vi "STM32.DAC.vi"(6 "FileName":string, 7 "CMD":enum16{"Sine", "File", "Close Output"}(ring), 8 "Error In":errorcluster, 9 "AMP":u8, 10 "FREQ":u16, 11 "VISA_USB":refnum<visa-resource-name>) -> (0 "Error Out":errorcluster, 1 "Points":i32, 2 "命令数":u32, 3 "CMD List":string[](array[string]))   [LabVIEW 2012, in "Lib_UEL.ATE.lvlib" / "STM32-CoreBD.lvlib"]
uses:
  STM32-CoreBD.lvlib
  <vilib>/regexp/Match Regular Expression.xnode
panel:
  # "Version History\nV01,2014-4-30, 初始版本."
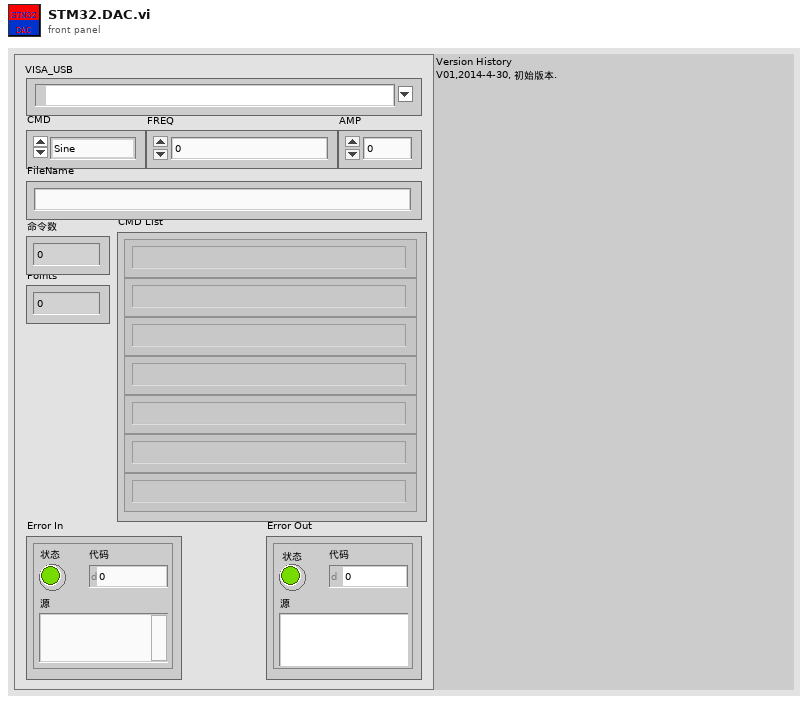
[diagram p1: front panel]
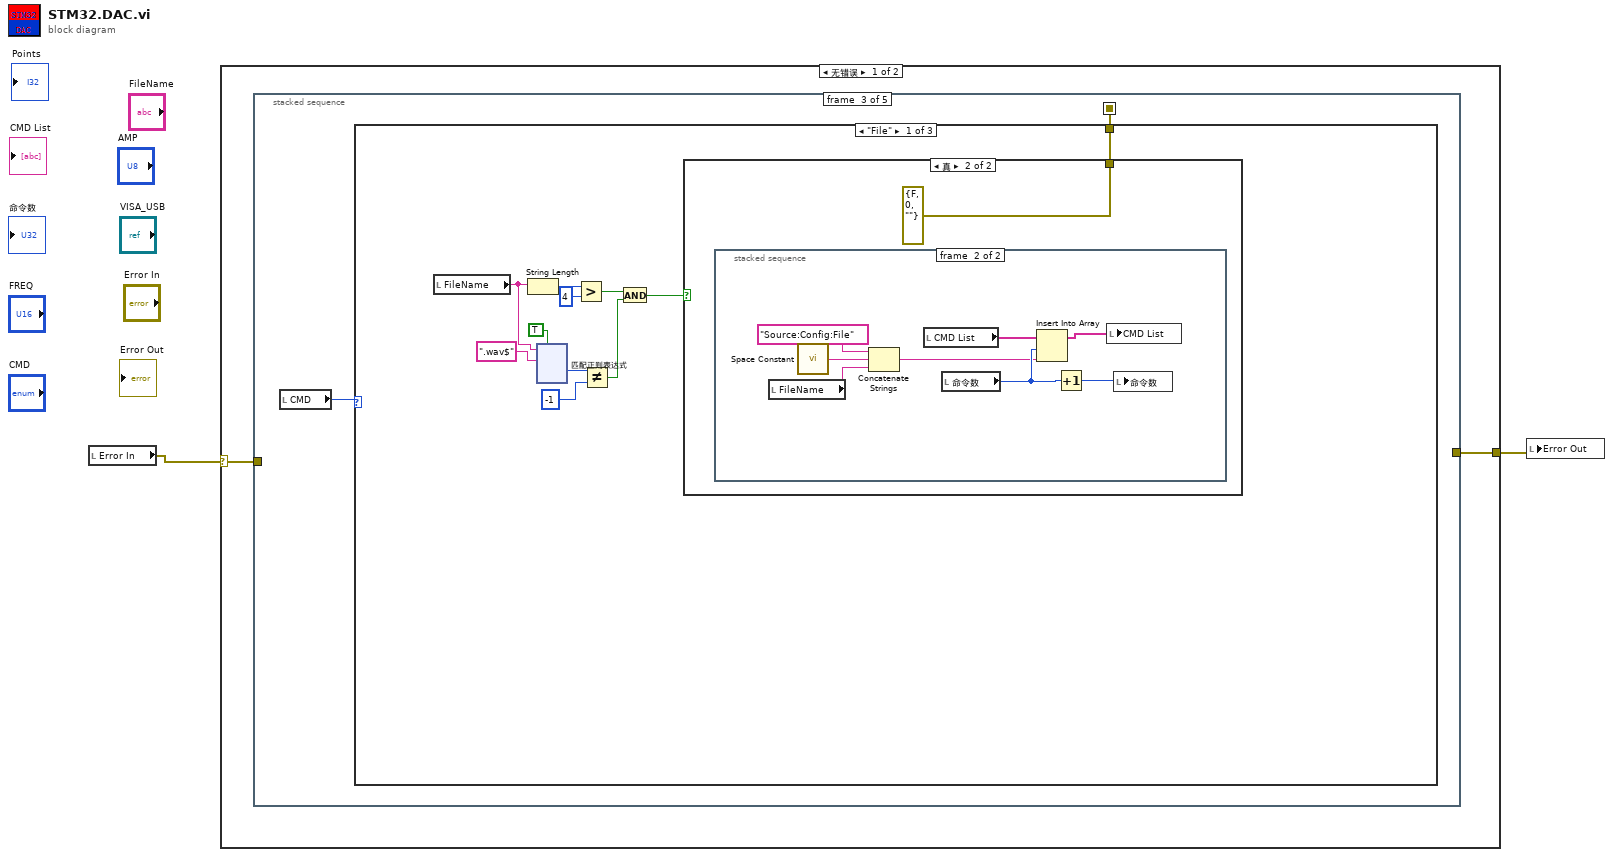
[diagram p0: block diagram]
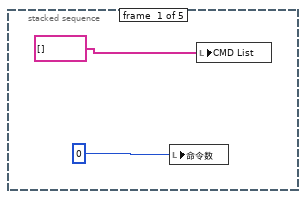
[diagram p2: hidden frame]
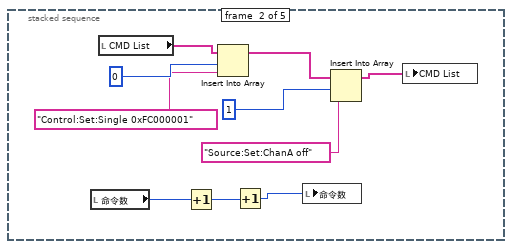
[diagram p3: hidden frame]
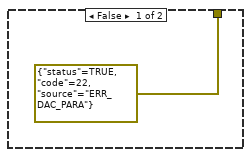
[diagram p4: hidden frame]
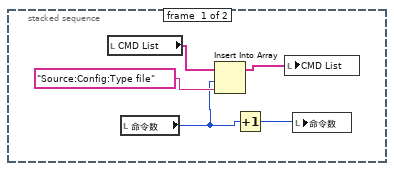
[diagram p5: hidden frame]
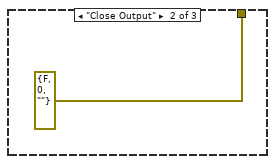
[diagram p6: hidden frame]
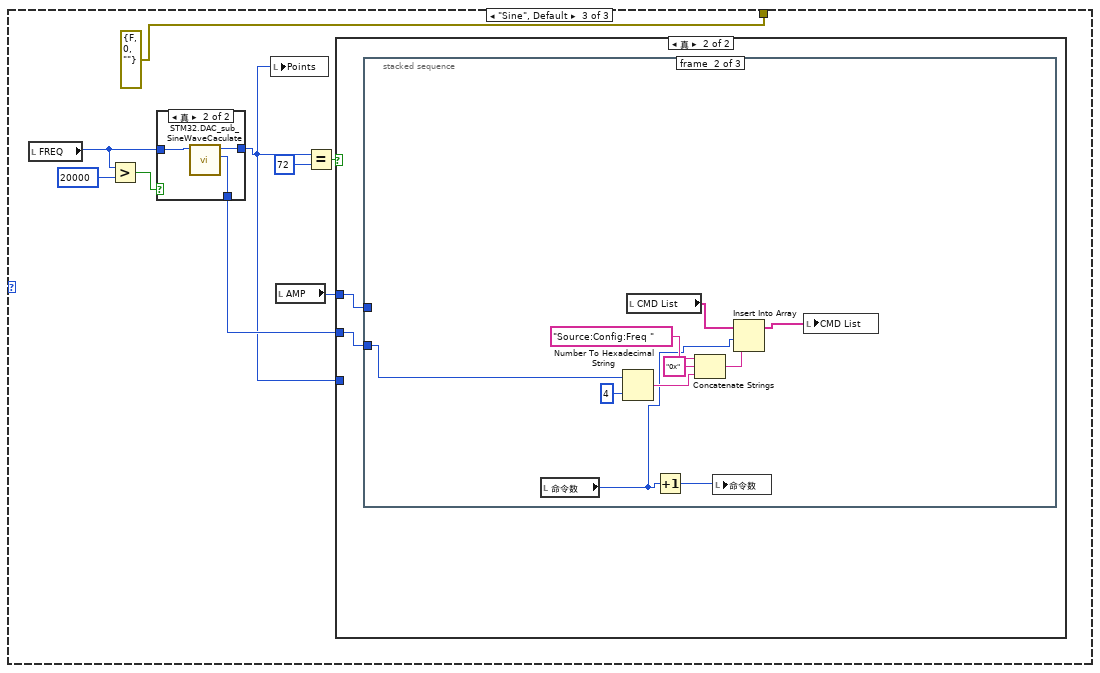
[diagram p7: hidden frame]
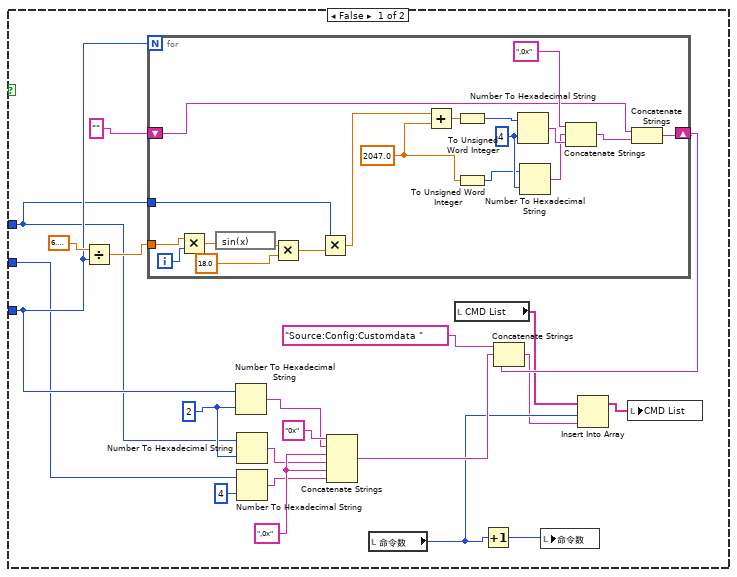
[diagram p8: hidden frame]
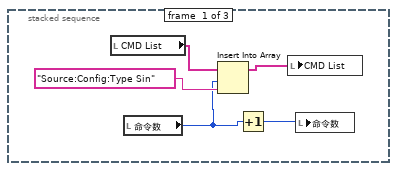
[diagram p9: hidden frame]
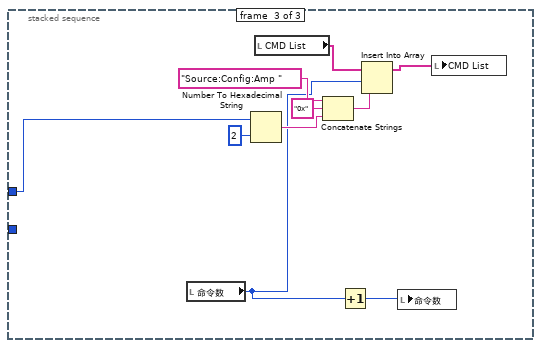
[diagram p10: hidden frame]
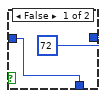
[diagram p11: hidden frame]
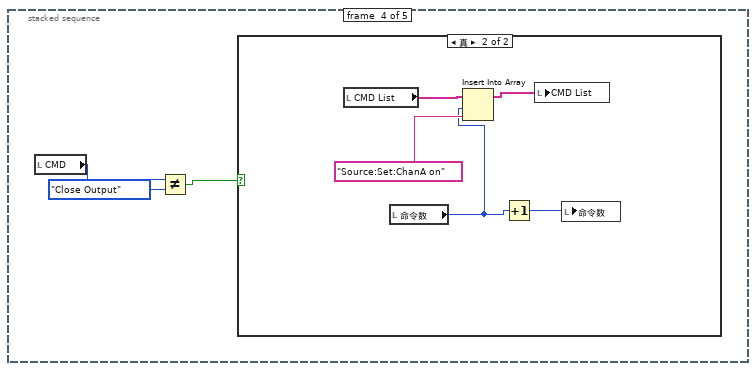
[diagram p12: hidden frame]
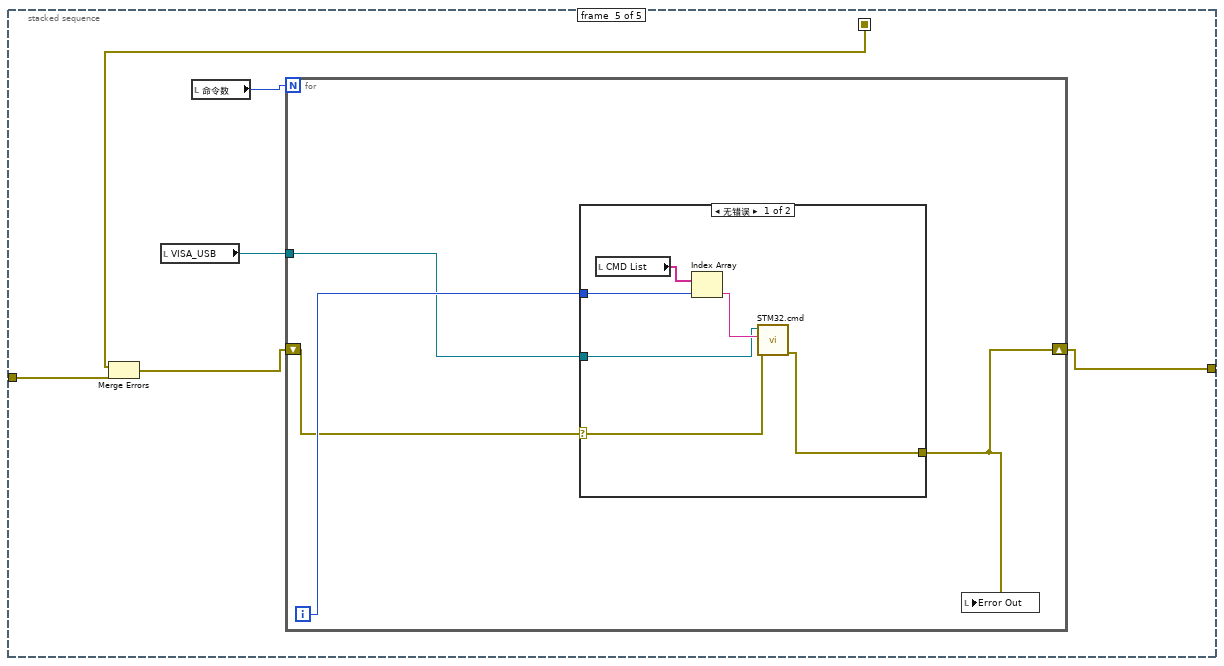
[diagram p14: hidden frame]
diagram:
  n1 = local read "Error In"() -> (w2:errorcluster)
  n2 = case shown="无错误" w2 {
    selector: w2 -> [w4 w263]
    tunnel: [w3 w263] -> w1
    frame No Error {
      n3 = stacked-sequence {
        seq-local: [_ _ w17 _ _] -> [_ _ _ _ w246]
        tunnel: w4 -> [_ _ _ _ w248]
        tunnel: [_ _ _ _ w249] -> w3
        frame #0 {
          n4 = local write "命令数"(0) -> ()
          n5 = local write "CMD List"(string[] []) -> ()
        }
        frame #1 {
          n6 = local read "命令数"() -> (w8:u32)
          n7 = local read "CMD List"() -> (w13:string[])
          n8 = Increment(x=w8) -> (x+1=w9:u32)
          n9 = Insert Into Array(array=w13, index=0 ("索引"), new element="Control:Set:Single 0xFC000001" ("新元素/子数组")) -> (w7:string[])
          n10 = Increment(x=w9) -> (x+1=w10:u32)
          n11 = local write "命令数"(w10) -> ()
          n12 = Insert Into Array(array=w7, index=1 ("索引"), new element="Source:Set:ChanA off" ("新元素/子数组")) -> (w14:string[])
          n13 = local write "CMD List"(w14) -> ()
        }
        frame #2 {
          n14 = local read "CMD"() -> (w18:enum16{"Sine", "File", "Close Output"})
          n15 = case shown="\"File\"" w18 {
            tunnel: [w19 errorcluster {"status"=FALSE, "code"=0, "source"=""} ("error IO") errorcluster {"status"=FALSE, "code"=0, "source"=""} ("error IO")] -> w17
            frame "File" {
              n16 = local read "FileName"() -> (w27:string)
              n17 = String Length(string=w27) -> (length=w29:i32)
              n18 = xnode "匹配正则表达式"("输入字符串"=w27, "正则表达式"=".wav$" ("搜索字符串"), "忽略大小写？(F)"=TRUE) -> ("匹配后偏移量"=w24:i32)  [unwired: 3 in, 4 out]
              n19 = Greater?(x=w29, y=4) -> (0:w22:bool)
              n20 = Not Equal?(x=w24, y=-1) -> (x != y?=w21:bool)
              n21 = And(x=w22, y=w21) -> (x .and. y?=w20:bool)
              n22 = case shown="真" w20 {
                tunnel: [errorcluster {"status"=TRUE, "code"=22, "source"="ERR_DAC_PARA"} ("error IO") errorcluster {"status"=FALSE, "code"=0, "source"=""} ("error IO")] -> w19
                frame False {
                }
                frame True {
                  n23 = stacked-sequence {
                    frame #0 {
                      n24 = local read "CMD List"() -> (w35:string[])
                      n25 = local read "命令数"() -> (w32:u32)
                      n26 = Insert Into Array(array=w35, index=w32, new element="Source:Config:Type file") -> (w34:string[])
                      n27 = Increment(x=w32) -> (x+1=w33:u32)
                      n28 = local write "CMD List"(w34) -> ()
                      n29 = local write "命令数"(w33) -> ()
                    }
                    frame #1 {
                      n30 = local read "FileName"() -> (w38:string)
                      n31 = call <vilib>:"Space Constant.vi"() -> ("String"=w39:string)
                      n32 = Concatenate Strings("Source:Config:File", w39, w38) -> (w37:string)
                      n33 = local read "CMD List"() -> (w44:string[])
                      n34 = local read "命令数"() -> (w41:u32)
                      n35 = Insert Into Array(array=w44, index=w41, new element=w37) -> (w43:string[])
                      n36 = Increment(x=w41) -> (x+1=w42:u32)
                      n37 = local write "CMD List"(w43) -> ()
                      n38 = local write "命令数"(w42) -> ()
                    }
                  }
                }
              }
            }
            frame "Close Output" {
            }
            frame "Sine", Default {
              n39 = local read "FREQ"() -> (w161:u16)
              n40 = Greater?(x=w161, y=u16 20000) -> (0:w165:bool)
              n41 = case shown="真" w165 {
                tunnel: w161 -> [w233 w236]
                tunnel: [72 ("最优值") w237] -> w158
                tunnel: [w233 w235] -> w159
                frame False {
                }
                frame True {
                  n42 = call "STM32.DAC_sub_SineWaveCaculate.vi"("频率"=w236) -> ("调整后频率"=w235:u16, "最优值"=w237:i32)  [unwired: 9 in]
                }
              }
              n43 = local write "Points"(w158) -> ()
              n44 = local read "AMP"() -> (w160:u8)
              n45 = Equal?(x=w158, y=72) -> (x = y?=w162:bool)
              n46 = case shown="真" w162 {
                tunnel: w159 -> [w167 w207]
                tunnel: w160 -> [w166 w206]
                tunnel: w158 -> [w168 _]
                frame False {
                  w186 = ",0x"
                  w180 = i16 2 ("宽度(-)")
                  n47 = Divide(x=6.283185307179586, y=w168) -> (x/y=w177:dbl)
                  n48 = for {
                    N: w168 -> [_]
                    tunnel: w177 -> [w204]
                    tunnel: w166 -> [w198]
                    shift-right: [w191] -> w176
                    shift-left: "" -> [w190]
                    i -> [w205]
                    w187 = 2047.0 ("y")
                    w196 = i16 4 ("宽度(-)")
                    n49 = Multiply(x=w204, y=w205) -> (x*y=w200:dbl)
                    n50 = expression code="sin(x)"(w200) -> (w199:dbl)
                    n51 = Multiply(x=w199, y=18.0) -> (x*y=w202:dbl)
                    n52 = Multiply(x=w198, y=w202) -> (x*y=w197:dbl)
                    n53 = Add(x=w197, y=w187) -> (x+y=w201:dbl)
                    n54 = To Unsigned Word Integer(number=w201) -> (unsigned 16bit integer=w194:u16)
                    n55 = To Unsigned Word Integer(number=w187) -> (unsigned 16bit integer=w195:u16)
                    n56 = Number To Hexadecimal String(1:w196, 2:w194) -> (0:w189:string)
                    n57 = Number To Hexadecimal String(1:w196, 2:w195) -> (0:w188:string)
                    n58 = Concatenate Strings(",0x", w188, w189) -> (w192:string)
                    n59 = Concatenate Strings(w190, w192) -> (w191:string)
                  }
                  n60 = Number To Hexadecimal String(1:w180, 2:w168) -> (0:w182:string)
                  n61 = Number To Hexadecimal String(1:w180, 2:w166) -> (0:w184:string)
                  n62 = Number To Hexadecimal String(1:i16 4 ("宽度(-)"), 2:w167) -> (0:w185:string)
                  n63 = Concatenate Strings("0x", w182, w186, w184, w186, w185) -> (w175:string)
                  n64 = local read "命令数"() -> (w171:u32)
                  n65 = local read "CMD List"() -> (w172:string[])
                  n66 = Increment(x=w171) -> (x+1=w173:u32)
                  n67 = Concatenate Strings("Source:Config:Customdata ", w175, w176) -> (w170:string)
                  n68 = local write "命令数"(w173) -> ()
                  n69 = Insert Into Array(array=w172, index=w171, new element=w170) -> (w169:string[])
                  n70 = local write "CMD List"(w169) -> ()
                }
                frame True {
                  n71 = stacked-sequence {
                    tunnel: w207 -> [_ w215 _]
                    tunnel: w206 -> [_ _ w223]
                    frame #0 {
                      n72 = local read "CMD List"() -> (w211:string[])
                      n73 = local read "命令数"() -> (w208:u32)
                      n74 = Insert Into Array(array=w211, index=w208, new element="Source:Config:Type Sin") -> (w210:string[])
                      n75 = Increment(x=w208) -> (x+1=w209:u32)
                      n76 = local write "CMD List"(w210) -> ()
                      n77 = local write "命令数"(w209) -> ()
                    }
                    frame #1 {
                      n78 = local read "命令数"() -> (w213:u32)
                      n79 = Number To Hexadecimal String(1:i16 4 ("宽度(-)"), 2:w215) -> (0:w216:string)
                      n80 = local read "CMD List"() -> (w221:string[])
                      n81 = Increment(x=w213) -> (x+1=w214:u32)
                      n82 = Concatenate Strings("Source:Config:Freq ", "0x" ("字符串"), w216) -> (w219:string)
                      n83 = local write "命令数"(w214) -> ()
                      n84 = Insert Into Array(array=w221, index=w213, new element=w219) -> (w222:string[])
                      n85 = local write "CMD List"(w222) -> ()
                    }
                    frame #2 {
                      n86 = local read "命令数"() -> (w224:u32)
                      n87 = Number To Hexadecimal String(1:i16 2 ("宽度(-)"), 2:w223) -> (0:w232:string)
                      n88 = local read "CMD List"() -> (w227:string[])
                      n89 = Concatenate Strings("Source:Config:Amp ", "0x" ("字符串"), w232) -> (w229:string)
                      n90 = Increment(x=w224) -> (x+1=w225:u32)
                      n91 = Insert Into Array(array=w227, index=w224, new element=w229) -> (w226:string[])
                      n92 = local write "命令数"(w225) -> ()
                      n93 = local write "CMD List"(w226) -> ()
                    }
                  }
                }
              }
            }
          }
        }
        frame #3 {
          n94 = local read "CMD"() -> (w240:enum16{"Sine", "File", "Close Output"})
          n95 = Not Equal?(x=w240, y=enum16{"Sine", "File", "Close Output"}."Close Output") -> (x != y?=w238:bool)
          n96 = case shown="真" w238 {
            frame False {
            }
            frame True {
              n97 = local read "CMD List"() -> (w244:string[])
              n98 = local read "命令数"() -> (w241:u32)
              n99 = Insert Into Array(array=w244, index=w241, new element="Source:Set:ChanA on" ("新元素/子数组")) -> (w243:string[])
              n100 = Increment(x=w241) -> (x+1=w242:u32)
              n101 = local write "CMD List"(w243) -> ()
              n102 = local write "命令数"(w242) -> ()
            }
          }
        }
        frame #4 {
          n103 = Merge Errors(w246, w248) -> (w247:errorcluster)
          n104 = local read "VISA_USB"() -> (w250:refnum<visa-resource-name>)
          n105 = local read "命令数"() -> (w251:u32)
          n106 = for {
            N: w251 -> [_]
            tunnel: w250 -> [w253]
            shift-right: [w252] -> w249
            shift-left: w247 -> [w254]
            i -> [w255]
            n107 = case shown="无错误" w254 {
              selector: w254 -> [w257 w262]
              tunnel: w255 -> [w260 _]
              tunnel: w253 -> [w258 _]
              tunnel: [w256 w262] -> w252
              frame No Error {
                n108 = local read "CMD List"() -> (w261:string[])
                n109 = Index Array(array=w261, index=w260) -> (element=w259:string)
                n110 = call "STM32.cmd.vi"("Error In"=w257, "命令"=w259, "VISA资源输入"=w258) -> ("Error Out"=w256:errorcluster)  [unwired: 5 in, 3 out]
              }
              frame Error {
              }
            }
            n111 = local write "Error Out"(w252) -> ()
          }
        }
      }
    }
    frame Error {
    }
  }
  n112 = local write "Error Out"(w1) -> ()
